vi "Close Error Handles.vi"(8 "error in":errorcluster, 11 "Error Handling Cluster":T1) -> (0 "error out":errorcluster)   [LabVIEW 2013, in "OPC UA Client Engine.lvlib" / "Error Handling API.lvlib"]
uses:
  Error Handling API.lvlib
  Controls/Error Handling Cluster.ctl
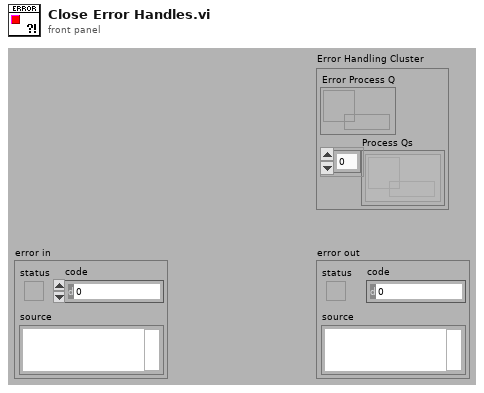
[diagram p1: front panel]
types:
  T1 = typedef "OPC UA Client Engine.lvlib/Error Handling API.lvlib/Error Handling Cluster.ctl" = cluster{"Error Process Q":refnum<queue>, "Process Qs":refnum<queue>[]}
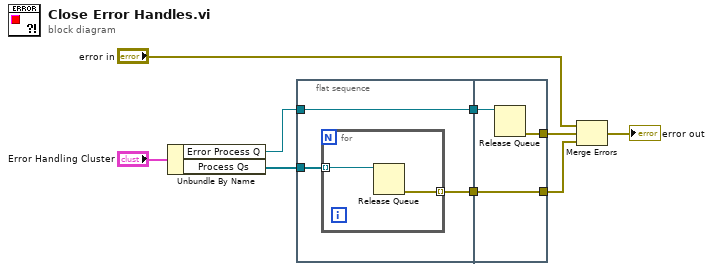
[diagram p0: block diagram]
diagram:
  n1 = Unbundle By Name("Error Handling Cluster") -> ("Error Process Q"=w6:refnum<queue>, "Process Qs"=w8:refnum<queue>[])
  n2 = flat-sequence {
    tunnel: w8 -> [w12]
    tunnel: [w11] -> w7
    tunnel: w6 -> [w11]
    tunnel: [w10] -> w3
    tunnel: w7 -> [w17]
    tunnel: [w16] -> w5
    tunnel: [w15] -> w4
    tunnel: w3 -> [w15]
    frame #0 {
      n3 = for {
        tunnel: w12 -> [w14] mode=indexing
        tunnel: [w13] -> w10 mode=indexing
        n4 = Release Queue(queue=w14) -> (error out=w13:errorcluster)  [unwired: 2 in, 2 out]
      }
    }
    frame #1 {
      n5 = Release Queue(queue=w17) -> (error out=w16:errorcluster)  [unwired: 2 in, 2 out]
    }
  }
  n6 = Merge Errors("error in", w5, w4) -> (→"error out":errorcluster)
